vi "__enterSetPoint.vi"(6 "error in (no error)":errorcluster, 7 "ActualSP":dbl=1000.0 min=0.0 max=1000000.0 step=0.1 format="%.2f") -> (0 "error out":errorcluster, 1 "NuevoSP 2":dbl min=0.0 max=999.9 step=0.1 format="%.2f", 3 "Cancelled?":bool)   [LabVIEW 2017]
doc: "Use this template to create a dialog box. This template polls the state of the buttons on the front panel and does not use events. Use the Dialog Using Events template (not available in Base package) to create a dialog box with event handling."
panel:
  in  "NuevoSP":dbl format="%.2f"
  in  "Cancel":bool
  in  "OK":bool
  # "Introduce el nuevo valor del flujo:"
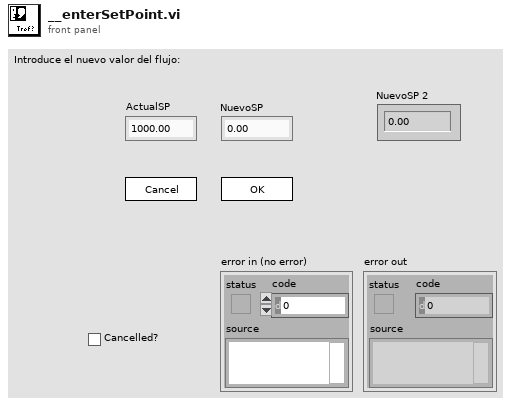
[diagram p1: front panel]
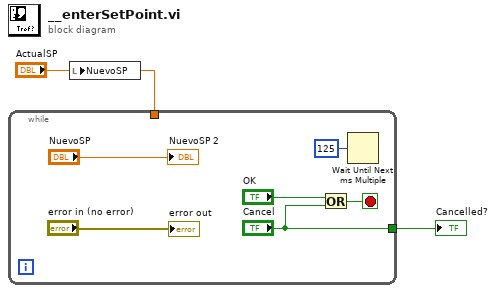
[diagram p0: block diagram]
diagram:
  n1 = while {
    tunnel: ["Cancel"] -> w2
    tunnel: "ActualSP" -> [_]
    stop <- w7 stop-if-true
    n2 = Or(x="OK", y="Cancel") -> (x .or. y?=w7:bool)
    n3 = Wait Until Next ms Multiple(millisecond multiple=u32 125) -> ()  [unwired: 1 out]
    "error out" <- "error in (no error)"
    "NuevoSP 2" <- "NuevoSP"
  }
  "Cancelled?" <- w2
  n4 = local write "NuevoSP"("ActualSP") -> ()
